vi "Check and Generate Path to Octave Executable.vi"(8 "error in (no error)":errorcluster, 11 "octave executable file or directory with executable":path=path "C:/Octave/Octave-4.0.0/bin") -> (0 "error out":errorcluster, 3 "path to exe":path)   [LabVIEW 2020, in "GOLPI library.lvlib"]
doc: "Checks path provided by user if exists. If file, consider it as Octave executable. If directory, try to look for octave-cli.exe or octave.exe. Return path to Octave executable or generate an error."
uses:
  GOLPI library.lvlib
  Type Definitions/Custom Error Codes Enum Type Def.vi
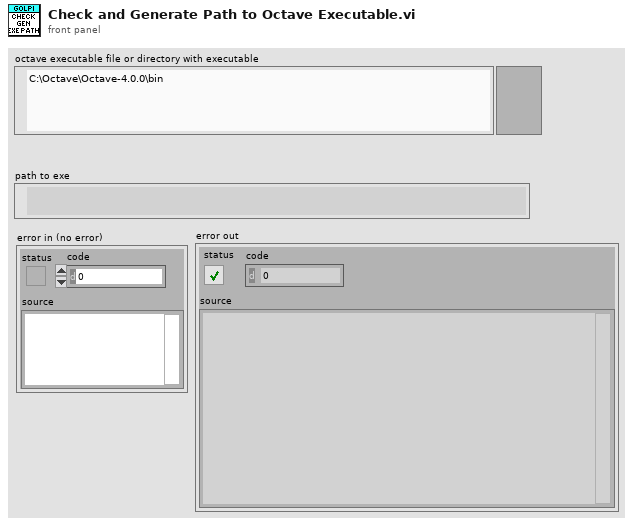
[diagram p1: front panel]
types:
  T1 = typedef "GOLPI library.lvlib/Custom Error Codes Enum Type Def.vi" = enum16{"no error", "00 working directory PAR1 missing", "01 octave binary PAR1 missing", "02 octave report error PAR1", "03 empty output last cmd PAR1", "04 missing temporary file PAR1", "05 pwd PAR 1 not exist", "06 oct package not installed", "07 octave default binary missing", "10 var PAR1 not string, vect", "11 var PAR1 not num, scal, ~compl", "12 var PAR1 not num, scal, compl", "13 var PAR1 not num, vect, ~compl", "14 var PAR1 not num, vect, compl", "15 var PAR1 not num, mat, ~compl", "16 var PAR1 not num, mat, ~compl", "30 read timeout", "60 bitstream transport failed", "61 bitstream decode error PAR1", "62 bitstream cannot be set", "70 struct transfer not possible", "80 struct: cluster elem. PAR1 not implem.", "81 struct: structure field PAR1 not implem.", "82 struct: size mismatch of PAR1", "83 struct: type mismatch of PAR1", "98 internal error", "99 not finished", "90 Not supported in Matlab mode", "91 Matlab variable transfer error", "92 Matlab Script Error", "100 Variable Pipe Mode cannot be set"}
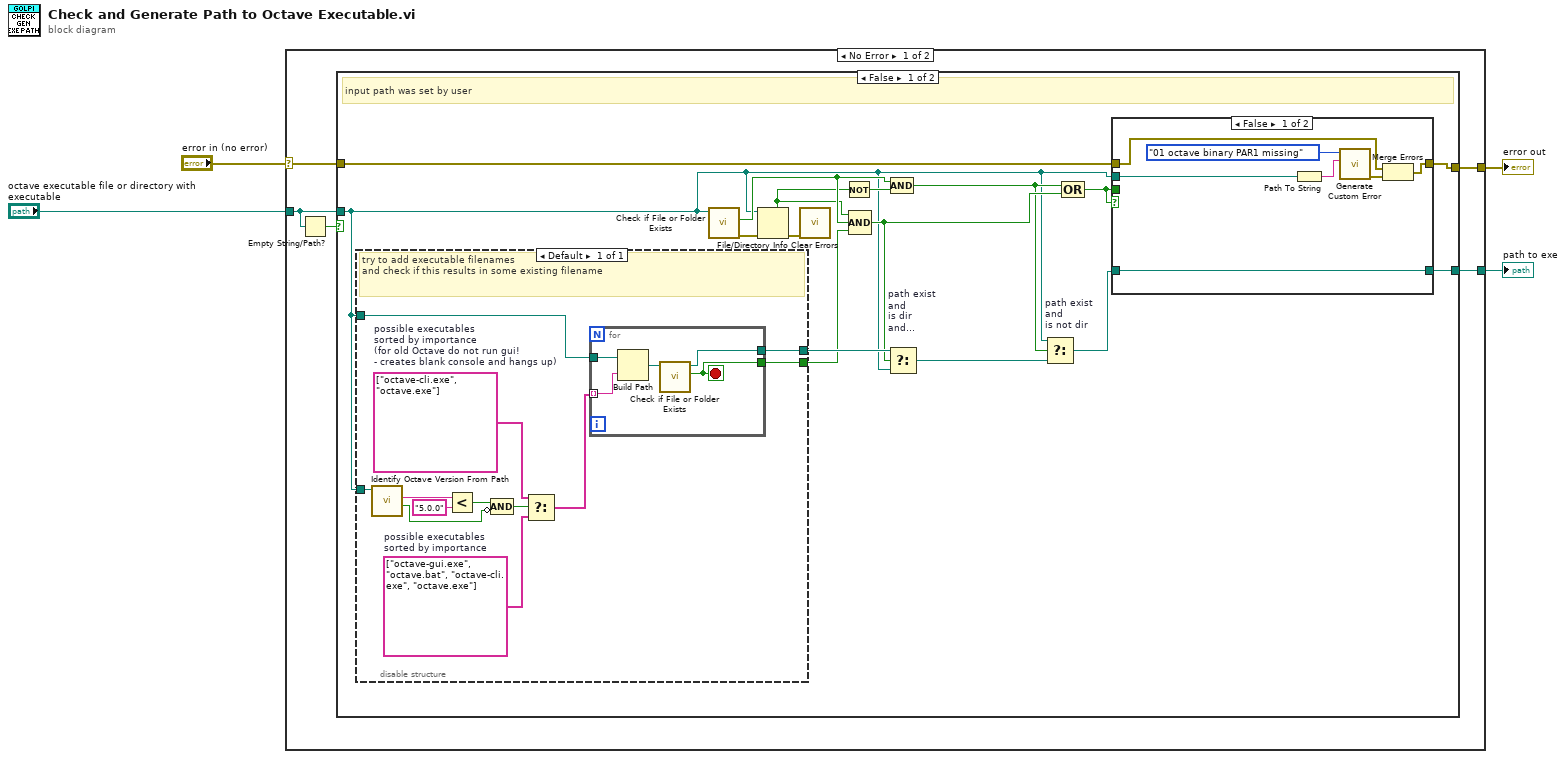
[diagram p0: block diagram]
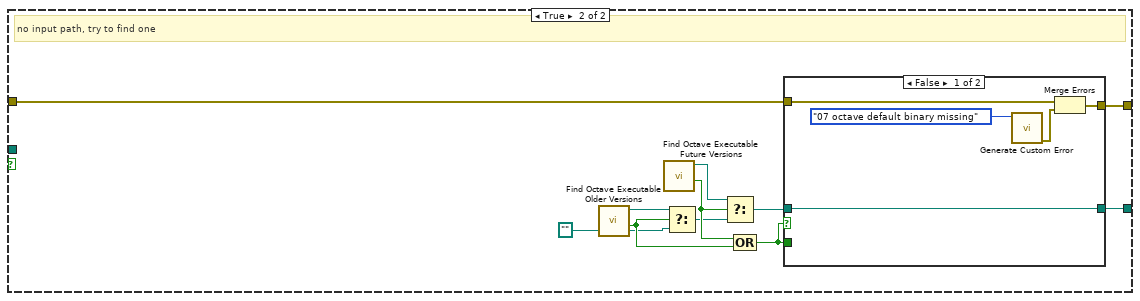
[diagram p3: hidden frame]
diagram:
  n1 = case shown="No Error" "error in (no error)" {
    selector: "error in (no error)" -> [w9 w71]
    tunnel: [w5 w71] -> w3
    tunnel: [w6 w70] -> w1
    tunnel: "octave executable file or directory with executable" -> [w8 w70]
    frame No Error {
      n2 = Empty String/Path?(string/path=w8) -> (empty?=w7:bool)
      n3 = case shown="False" w7 {
        tunnel: [w13 w55] -> w5
        tunnel: w9 -> [w14 w56]
        tunnel: [w11 w52] -> w6
        tunnel: w8 -> [w10 _]
        frame False {
          # "input path was set by user"
          n4 = disable-structure shown="Default" {
            disable-tunnel: [w37] -> w24
            disable-tunnel: [w36] -> w16
            disable-tunnel: w10 -> [w35]
            disable-tunnel: w10 -> [w34]
            frame Enabled {
              w28 = string[] ["octave-gui.exe", "octave.bat", "octave-cli.exe", "octave.exe"]  # possible executables sorted by importance
              w27 = string[] ["octave-cli.exe", "octave.exe"]  # possible executables sorted by importance (for old Octave do not run gui! - creates blank console and hangs up)
              # "try to add executable filenames\nand check if this results in some existing filename"
              n5 = call "Identify Octave Version From Path.vi"("Octave path (file or bin folder)"=w34) -> ("not identified"=w30:bool, "version string"=w33:string)  [unwired: 7 in, 2 out]
              n6 = Less?(x=w33, y="5.0.0") -> (x < y?=w31:bool)
              n7 = Compound Arithmetic op=AND(w31, invert w30) -> (w29:bool)
              n8 = Select(t=w27, s=w29, f=w28) -> (s? t:f=w26:string[])
              n9 = for {
                tunnel: w26 -> [w42] mode=indexing
                tunnel: w35 -> [w41]
                tunnel: [w39] -> w37
                tunnel: [w38] -> w36
                stop <- w38 stop-if-true
                n10 = Build Path(base path=w41, name or relative path=w42) -> (appended path=w40:path)
                n11 = call <vilib>:"Check if File or Folder Exists.vi"("path"=w40) -> ("file or folder exists?"=w38:bool, "dup path"=w39:path)  [unwired: 8 in, 1 out]
              }
            }
          }
          n12 = call <vilib>:"Check if File or Folder Exists.vi"("path"=w10) -> ("error out"=w25:errorcluster, "file or folder exists?"=w20:bool)  [unwired: 8 in, 1 out]
          n13 = File/Directory Info(path=w10, error in=w25) -> (directory=w19:bool, error out=w22:errorcluster)  [unwired: 5 out]
          n14 = call <vilib>:"Clear Errors.vi"("error in (no error)"=w22) -> ()  [unwired: 5 in, 2 out]
          n15 = Not(x=w19) -> (.not. x?=w21:bool)
          n16 = Compound Arithmetic op=AND(w19, w20, w16) -> (w18:bool)
          n17 = Select "path exist\nand\nis dir\nand\nexecutable found"(t=w24, s=w18, f=w10) -> (s? t:f=w23:path)
          n18 = Compound Arithmetic op=AND(w20, w21) -> (w17:bool)
          n19 = Select "path exist\nand\nis not dir"(t=w10, s=w17, f=w23) -> (s? t:f=w15:path)
          n20 = Compound Arithmetic op=OR(w17, w18) -> (w12:bool)
          n21 = case shown="False" w12 {
            tunnel: w15 -> [w44 w51]
            tunnel: w14 -> [w46 w50]
            tunnel: w12 -> [_ _]
            tunnel: [w45 w50] -> w13
            tunnel: [w44 w51] -> w11
            tunnel: w10 -> [w43 _]
            frame False {
              n22 = Path To String(path=w43) -> (string=w49:string)
              n23 = call "Generate Custom Error.vi"("PAR1"=w49, "GOLPI error"=Custom_Error_Codes_Enum_Type_Def.vi."01 octave binary PAR1 missing") -> ("error out"=w47:errorcluster)  [unwired: 9 in]
              n24 = Merge Errors(w46, w47) -> (w45:errorcluster)
            }
            frame True {
            }
          }
        }
        frame True {
          # "no input path, try to find one"
          n25 = call "Find Octave Executable Older Versions.vi"() -> ("Found executable?"=w62:bool, "Executable path"=w59:path)  [unwired: 10 in]
          n26 = call "Find Octave Executable Future Versions.vi"() -> ("Found executable?"=w61:bool, "Executable path"=w57:path)  [unwired: 10 in]
          n27 = Select(t=w59, s=w62, f=path "") -> (s? t:f=w60:path)
          n28 = Select(t=w57, s=w61, f=w60) -> (s? t:f=w53:path)
          n29 = Compound Arithmetic op=OR(w61, w62) -> (w54:bool)
          n30 = case shown="False" w54 {
            tunnel: w56 -> [w65 w68]
            tunnel: w54 -> [_ _]
            tunnel: [w64 w68] -> w55
            tunnel: [w63 w69] -> w52
            tunnel: w53 -> [w63 w69]
            frame False {
              n31 = call "Generate Custom Error.vi"("GOLPI error"=Custom_Error_Codes_Enum_Type_Def.vi."07 octave default binary missing") -> ("error out"=w66:errorcluster)  [unwired: 10 in]
              n32 = Merge Errors(w65, w66) -> (w64:errorcluster)
            }
            frame True {
            }
          }
        }
      }
    }
    frame Error {
    }
  }
  "error out" <- w3
  "path to exe" <- w1
